vi "MotorMultiWait.vi"(4 "Ok?":refnum<k4>[](array[refnum]), 9 "error out":errorcluster caption="error in (no error)") -> (6 "error in (no error)":errorcluster caption="error out")   [LabVIEW 2009]
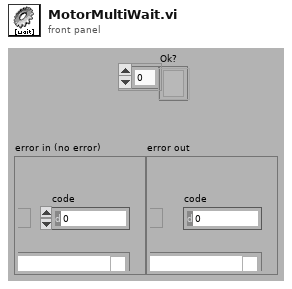
[diagram p1: front panel]
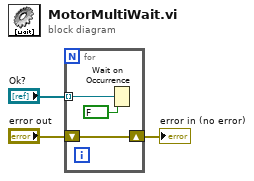
[diagram p0: block diagram]
diagram:
  n1 = for {
    tunnel: "Ok?" -> [w5] mode=indexing
    shift-right: [w6] -> w2
    shift-left: "error out" -> [w6]
    n2 = Wait on Occurrence(1:FALSE ("ignorer précédent (V)"), 2:w5) -> ()  [unwired: 2 out]
  }
  "error in (no error)" <- w2
